vi "Read File.vi"(8 "Error In":errorcluster, 11 "Mux File Path":path) -> (0 "Error Out":errorcluster, 3 "Mux Data Array":T1[](array[typedef]))   [LabVIEW 2013, in "MUX Custom Device.lvlib"]
uses:
  MUX Custom Device.lvlib
  SubVIs/Mux Data.ctl
  SubVIs/Relay Channel Data.ctl
  SubVIs/Relay Data.ctl
  SubVIs/Switch.ctl
  <vilib>/Utility/file.llb/Read From Spreadsheet File (string).vi
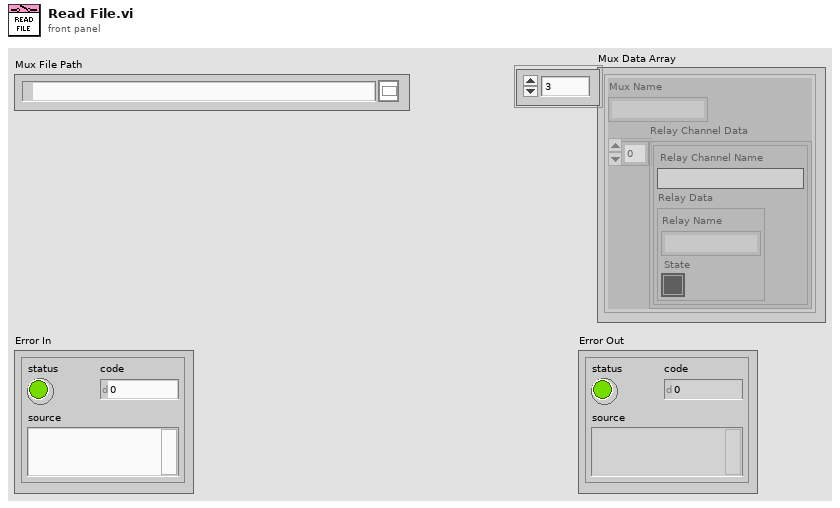
[diagram p1: front panel]
types:
  T1 = typedef "MUX Custom Device.lvlib/Mux Data.ctl" = cluster{"Mux Name":string, "Relay Channel Data":T2[]}
  T2 = typedef "MUX Custom Device.lvlib/Relay Channel Data.ctl" = cluster{"Relay Channel Name":string, "Relay Data":T3}
  T3 = typedef "MUX Custom Device.lvlib/Relay Data.ctl" = cluster{"Relay Name":string, "State":T4}
  T4 = typedef "MUX Custom Device.lvlib/Switch.ctl" = bool
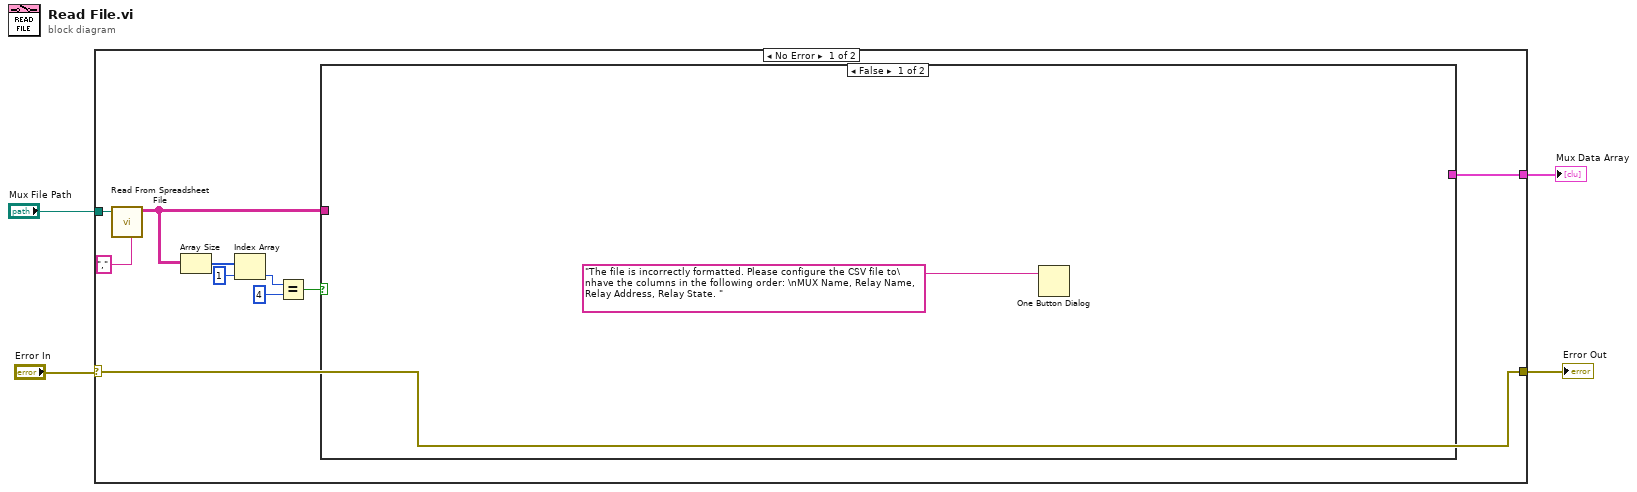
[diagram p0: block diagram]
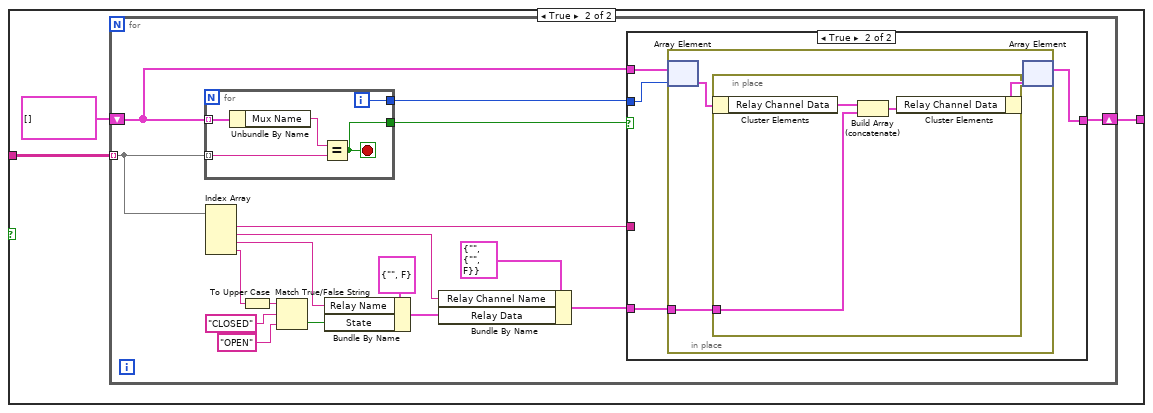
[diagram p2: hidden frame]
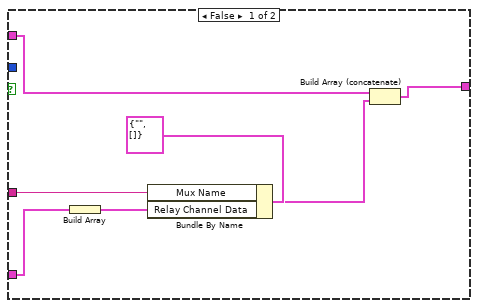
[diagram p3: hidden frame]
diagram:
  n1 = case shown="No Error" "Error In" {
    selector: "Error In" -> [w12 w58]
    tunnel: "Mux File Path" -> [w14 _]
    tunnel: [w13 _] -> w3
    tunnel: [w12 w58] -> w1
    frame No Error {
      n2 = call-poly <vilib>:"Read From Spreadsheet File.vi"("delimiter (\\t)"="," ("delimiter (\\t)"), "file path (dialog if empty)"=w14) -> ("all rows"=w11:string[][])  [unwired: 5 in, 4 out]
      n3 = Array Size(array=w11) -> (size(s)=w10:i32[])
      n4 = Index Array(array=w10, index=1) -> (element=w8:i32)
      n5 = Equal?(x=w8, y=4) -> (x = y?=w6:bool)
      n6 = case shown="False" w6 {
        tunnel: [_ w17] -> w13
        tunnel: w11 -> [_ w16]
        frame False {
          n7 = One Button Dialog(message="The file is incorrectly formatted. Please configure the CSV file to\nhave the columns in the following order: \nMUX Name, Relay Name, Relay Address, Relay State. ") -> ()  [unwired: 1 in, 1 out]
        }
        frame True {
          n8 = for {
            tunnel: w16 -> [w28] mode=indexing
            shift-right: [w32] -> w17
            shift-left: T1[] [] -> [w34]
            n9 = for {
              tunnel: w34 -> [w56] mode=indexing
              tunnel: w28 -> [w57] mode=indexing
              tunnel: [w54] -> w35
              tunnel: [w53] -> w33
              i -> [w53]
              stop <- w54 stop-if-true
              n10 = Unbundle By Name(w56) -> ("Mux Name"=w55:string)
              n11 = Equal?(x=w55, y=w57) -> (x = y?=w54:bool)
            }
            n12 = Index Array(array=w28) -> (element #1=w27:string, element #2=w20:string, element #3=w19:string, element #4=w24:string)  [unwired: 4 in]
            n13 = To Upper Case(1:w24) -> (0:w29:string)
            n14 = Match True/False String(2:"OPEN" ("false string"), 3:"CLOSED" ("true string"), 4:w29) -> (0:w25:bool)  [unwired: 1 out]
            n15 = Bundle By Name(cluster=T3 {"Relay Name"="", "State"=FALSE} ("Relay Data"), "Relay Name"=w19, "State"=w25) -> (w22:T3)
            n16 = Bundle By Name(cluster=T2 {"Relay Channel Name"="", "Relay Data"={"Relay Name"="", "State"=FALSE}} ("Relay Channel Data"), "Relay Channel Name"=w20, "Relay Data"=w22) -> (w21:T2)
            n17 = case shown="True" w35 {
              tunnel: w34 -> [w42 w46]
              tunnel: w27 -> [w39 _]
              tunnel: w33 -> [_ w45]
              tunnel: [w41 w44] -> w32
              tunnel: w21 -> [w38 w43]
              frame False {
                n18 = Build Array(w38) -> (w37:T2[])
                n19 = Bundle By Name(cluster=T1 {"Mux Name"="", "Relay Channel Data"=[]} ("Mux Data"), "Mux Name"=w39, "Relay Channel Data"=w37) -> (w36:T1)
                n20 = Build Array (concatenate)(w42, w36) -> (w41:T1[])
              }
              frame True {
                n21 = in-place {
                  in-place-border: w43 -> [w47]
                  n22 = in-place-array #1(w46, w45) -> (w49:T1)
                  n23 = in-place {
                    in-place-border: w47 -> [w50]
                    n24 = in-place-cluster #2(w49) -> ("Relay Channel Data"=w52:T2[])
                    n25 = Build Array (concatenate)(w52, w50) -> (w51:T2[])
                    n26 = in-place-cluster #2("Relay Channel Data"=w51) -> (w48:T1)
                  }
                  n27 = in-place-array #1(w48) -> (w44:T1[])  [unwired: 1 out]
                }
              }
            }
          }
        }
      }
    }
    frame Error {
    }
  }
  "Error Out" <- w1
  "Mux Data Array" <- w3
